vi "Msg Rescript.vi"() -> ()   [LabVIEW 2025]
uses:
  _Shared/_Shared.lvlib
  _Msg Rescript/_Msg Rescript/_Msg Rescript.lvclass
  _Shared/Panel/Panel.lvlib
  _Shared/Tree/Tree.lvlib
panel:
  out "Target":string
  in  "Tree":string(tree)
  in  "OK":bool
  # "Disclaimer: Please consider committing changes before AND after this action"
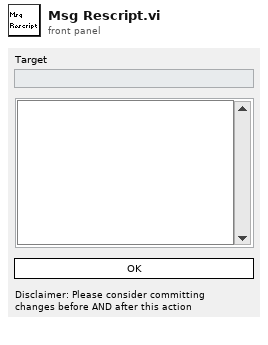
[diagram p1: front panel]
types:
  T1 = typedef "_Shared.lvlib/Type Name Library File Path.ctl" = map{T2, T3}
  T2 = typedef "_Shared.lvlib/Type.ctl" = enum16{"Actor", "Msg"}
  T3 = typedef "_Shared.lvlib/Name Library File Path.ctl" = map{string, path}
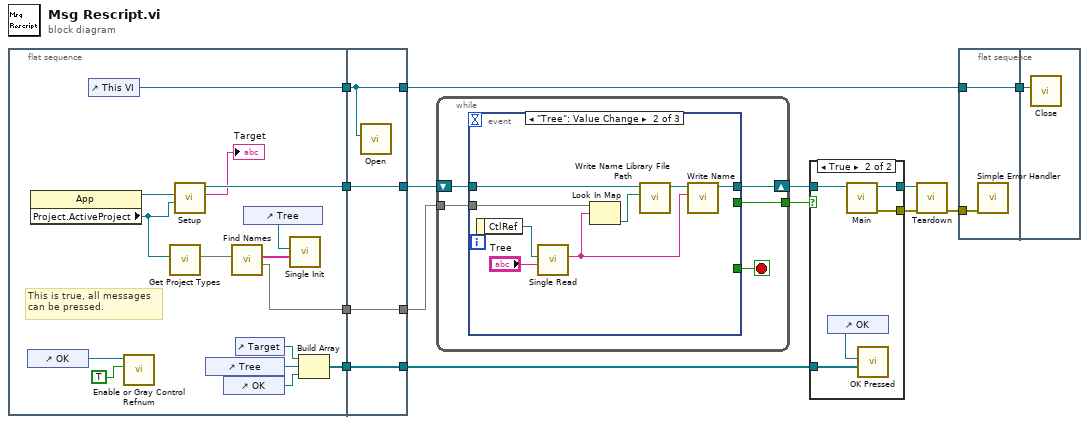
[diagram p0: block diagram]
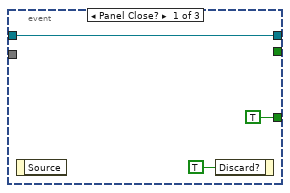
[diagram p2: hidden frame]
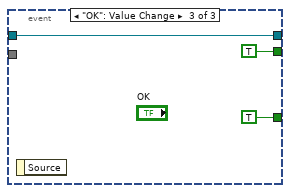
[diagram p3: hidden frame]
diagram:
  n1 = flat-sequence {
    tunnel: [w29] -> w10
    tunnel: [w18] -> w9
    tunnel: [w20] -> w6
    tunnel: [w27] -> w5
    tunnel: w10 -> [w33]
    tunnel: [w33] -> w2
    tunnel: [w32] -> w8
    tunnel: w9 -> [w32]
    tunnel: [w31] -> w7
    tunnel: w6 -> [w31]
    tunnel: [w30] -> w4
    tunnel: w5 -> [w30]
    frame #0 {
      # "This is true, all messages can be pressed."
      n2 = control-ref of="OK"() -> (w26:refnum<vi>)
      n3 = property class="App"() -> (reference out=w19:refnum<vi>, "Project.ActiveProject"=w17:refnum<vi>)  [unwired: 2 in, 1 out]
      n4 = control-ref of="This VI"() -> (w29:refnum<vi>)
      n5 = call <vilib>:"Enable or Gray Control Refnum.vi"("enable?"=TRUE, "Control in"=w26) -> ()  [unwired: 8 in, 2 out]
      n6 = call "Get Project Types.vi"("Project:Active Project"=w17) -> ("Type Name Library File Path"=w21:T1)  [unwired: 10 in]
      n7 = call "Setup.vi"("Active Project"=w17, "NI.LV.Dialog Instance"=w19) -> ("Target"=→"Target":string, "_Rescript Msg out"=w18:refnum<class "_Msg Rescript.lvclass">)  [unwired: 8 in]
      n8 = control-ref of="Tree"() -> (w23:refnum<vi>)
      n9 = control-ref of="OK"() -> (w28:refnum<vi>)
      n10 = call "Find Names.vi"("Type Name Library File Path"=w21) -> ("Name Library File Path"=w20:T3, "Names"=w22:string[])  [unwired: 9 in]
      n11 = control-ref of="Target"() -> (w15:refnum<vi>)
      n12 = control-ref of="Tree"() -> (w24:refnum<vi>)
      n13 = call "Single Init.vi"("Left Cell Strings"=w22, "Tree Ref"=w24) -> ()  [unwired: 10 in]
      n14 = Build Array(w15, w23, w28) -> (w27:refnum<vi>[])
    }
    frame #1 {
      n15 = call "Open.vi"("VI"=w33) -> ()  [unwired: 11 in]
    }
  }
  n16 = while {
    tunnel: [w38] -> w12
    shift-right: [w35] -> w11
    shift-left: w8 -> [w36]
    tunnel: w7 -> [w34]
    stop <- w37 stop-if-true
    n17 = event shown="[1] \"Tree\": Value Change" {
      selector: _ -> [_ _ _]
      dyn-events: _ -> [_ _ _]
      timeout: _ -> [_ _ _]
      tunnel: [_ _ TRUE ("Rename 2")] -> w38
      tunnel: [TRUE _ TRUE] -> w37
      tunnel: w36 -> [w39 w47 w52]
      tunnel: [w39 w42 w52] -> w35
      tunnel: w34 -> [_ w49 _]
      event Panel Close? {
        n18 = event-data() -> ()  [unwired: 1 in, 1 out]
        n19 = event-data("Discard?"=TRUE) -> ()  [unwired: 1 in, 1 out]
      }
      event "Tree": Value Change {
        n20 = event-data() -> ("CtlRef"=w45:refnum<vi>)  [unwired: 1 in]
        n21 = call "Single Read.vi"("Tree"="Tree", "Tree Ref"=w45) -> ("Name"=w43:string)  [unwired: 9 in]
        n22 = Look In Map(map=w49, key=w43) -> (value=w48:path)  [unwired: 1 in, 1 out]
        n23 = call "Write Name Library File Path.vi"("Name Library File Path"=w48, "_Rescript Msg in"=w47) -> ("_Rescript Msg out"=w46:refnum<class "_Msg Rescript.lvclass">)  [unwired: 9 in]
        n24 = call "Write Name.vi"("Name"=w43, "_Rescript Msg in"=w46) -> ("_Rescript Msg out"=w42:refnum<class "_Msg Rescript.lvclass">)  [unwired: 9 in]
      }
      event "OK": Value Change {
        n25 = event-data() -> ()  [unwired: 1 in, 1 out]
      }
    }
  }
  n26 = case shown="True" w12 {
    tunnel: w11 -> [w53 w58]
    tunnel: [w53 w57] -> w14
    tunnel: w4 -> [_ w55]
    tunnel: [_ w56] -> w13
    frame False {
    }
    frame True {
      n27 = control-ref of="OK"() -> (w54:refnum<vi>)
      n28 = call "Main.vi"("_Rescript Msg in"=w58) -> ("error out"=w56:errorcluster, "_Rescript Msg out"=w57:refnum<class "_Msg Rescript.lvclass">)  [unwired: 9 in]
      n29 = call "OK Pressed.vi"("Controls in"=w55, "OK Ref"=w54) -> ()  [unwired: 10 in]
    }
  }
  n30 = call "Teardown.vi"("error in"=w13, "_Rescript Msg in"=w14) -> ("error out"=w1:errorcluster)  [unwired: 9 in]
  n31 = flat-sequence {
    tunnel: w1 -> [w60]
    tunnel: w2 -> [w59]
    tunnel: [w59] -> w3
    tunnel: w3 -> [w61]
    frame #0 {
      n32 = call <vilib>:"Simple Error Handler.vi"("error in (no error)"=w60) -> ()  [unwired: 4 in, 5 out]
    }
    frame #1 {
      n33 = call "Close.vi"("VI"=w61) -> ()  [unwired: 11 in]
    }
  }
